vi "Test-Control-Panel.vi"() -> ()   [LabVIEW 2021]
uses:
  Global-Var-Simulator.vi
  Global-Var-OperService.vi
  Global-Var-ControlPanel.vi
panel:
  out "is_simulator_on":bool
  in  "all_alarm_delete_btn":bool
  in  "start_sim":bool
  in  "stop_sim":bool
  in  "shiner_level_ind_L":dbl
  in  "soap_level_ind_L":dbl
  in  "water_level_ind_L":dbl
  in  "download_values_button":bool
  in  "send_values_btn":bool
  in  "process_stop_btn":bool
  in  "fill_shiner_tank_btn":bool
  in  "fill_soap_tank_btn":bool
  in  "fill_water_tank_btn":bool
  out "low_shiner_level_alarm_ind":bool
  out "low_soap_level_alarm_ind":bool
  out "low_water_level_alarm_ind":bool
  out "broken_nozzle_stance_1_alarm_ind":bool
  out "high_temp_tank_1_alarm_ind":bool
  out "high_press_tank_1_alarm_ind":bool
  out "pump_clogged_alarm_ind":bool
  in  "broken_nozzle_stance_1_alarm_btn":bool
  in  "high_temperature_tank_1_alarm_btn":bool
  in  "high_pressure_tank_1_alarm_btn":bool
  in  "pump_clogged_alarm_btn":bool
  out "shiner_tank_L":dbl(slide) scale=0.0..500.0
  out "soap_tank_L":dbl(slide) scale=0.0..500.0
  out "water_tank_L":dbl(slide) scale=0.0..500.0
  # "ON/OFF"
  # "Tank control section"
  # "Alarms control\nand indication"
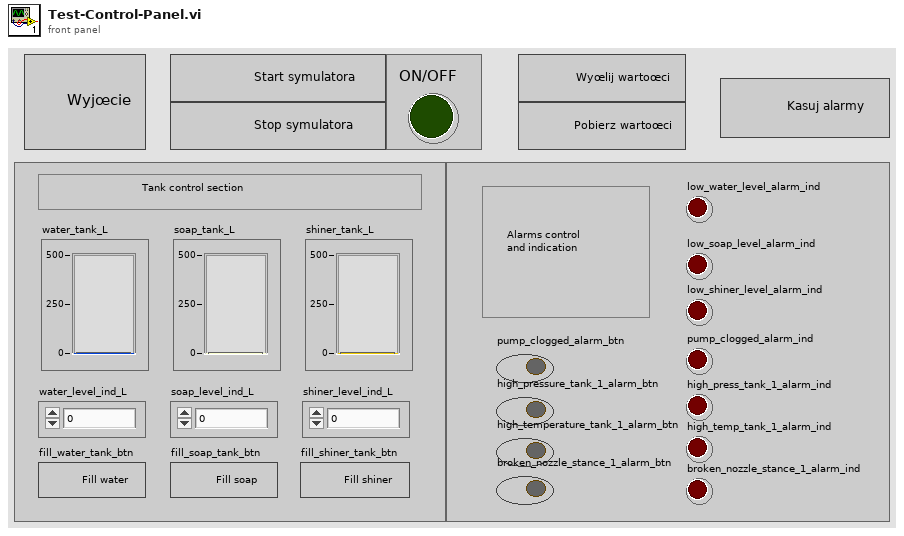
[diagram p1: front panel]
types:
  T1 = enum32{"Invalid", "Standard", "Closed", "Hidden", "Minimized", "Maximized"}
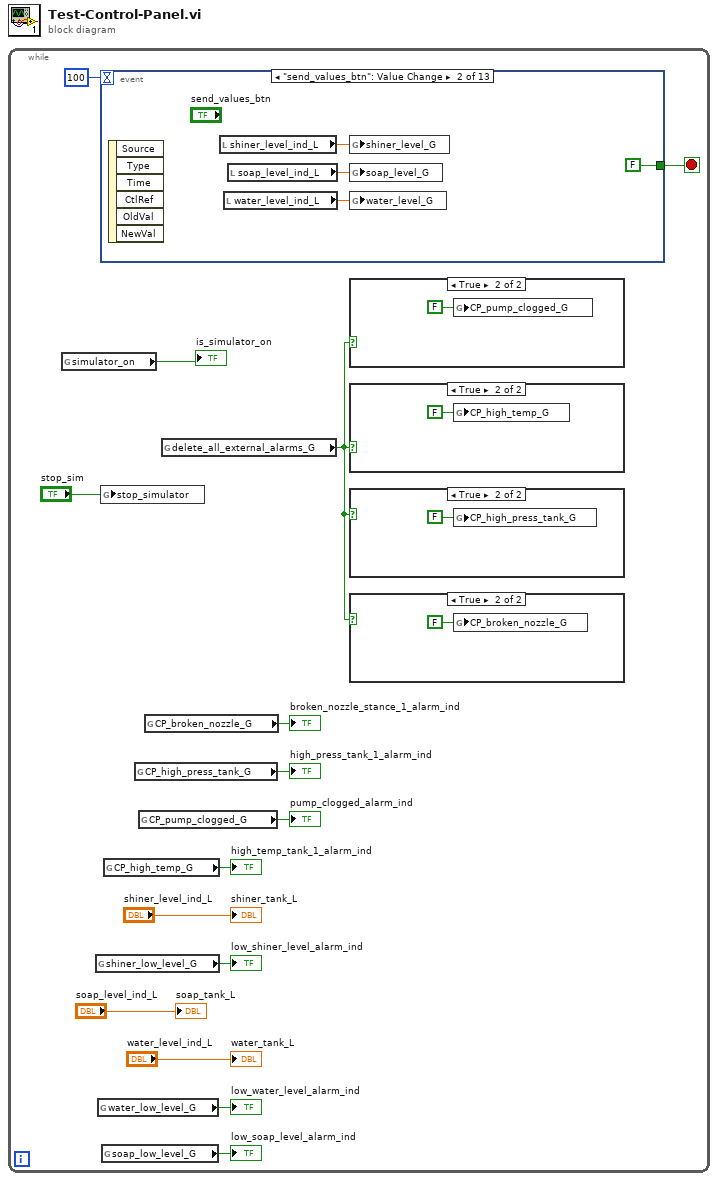
[diagram p0: block diagram]
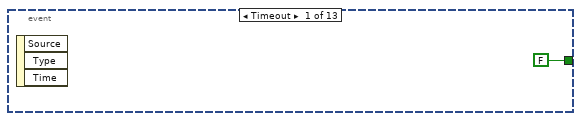
[diagram p6: hidden frame]
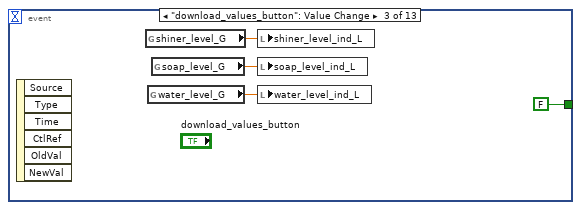
[diagram p7: hidden frame]
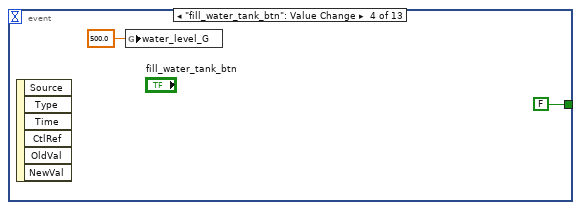
[diagram p8: hidden frame]
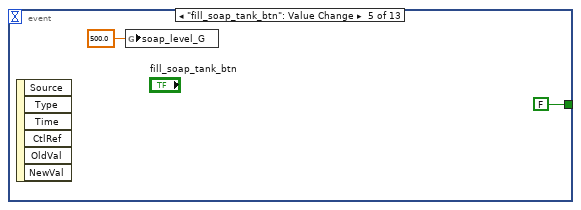
[diagram p9: hidden frame]
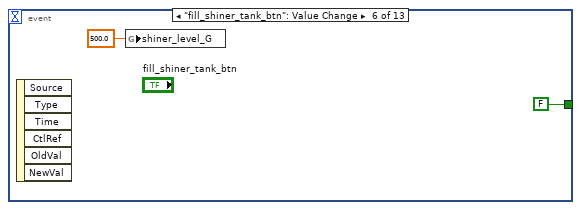
[diagram p10: hidden frame]
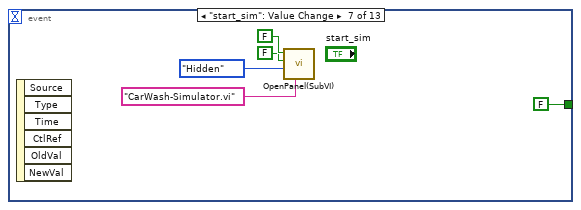
[diagram p11: hidden frame]
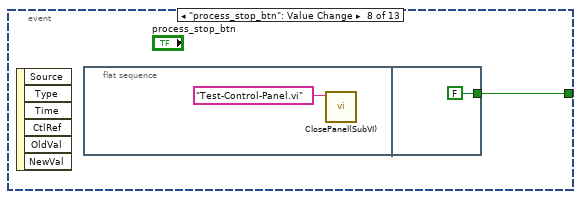
[diagram p12: hidden frame]
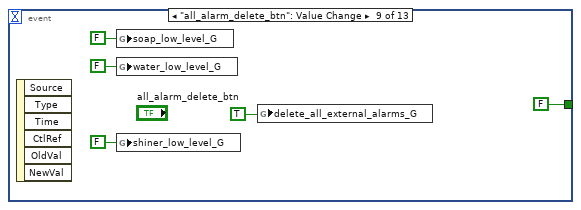
[diagram p13: hidden frame]
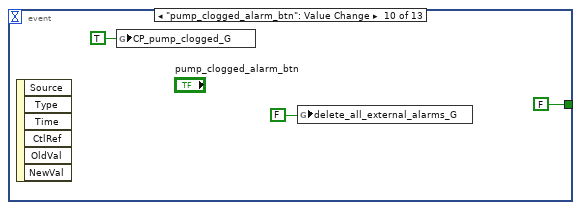
[diagram p14: hidden frame]
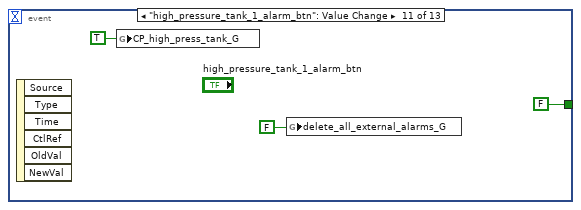
[diagram p15: hidden frame]
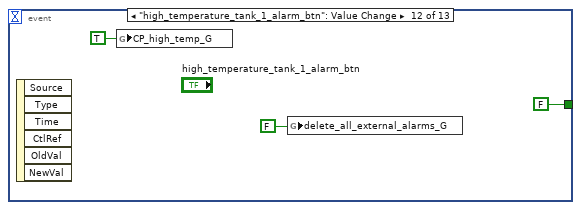
[diagram p16: hidden frame]
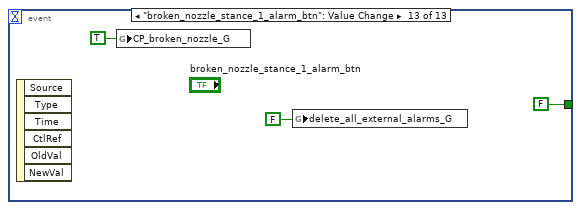
[diagram p17: hidden frame]
diagram:
  n1 = while {
    stop <- w10 stop-if-true
    n2 = global read "Global-Var-Simulator.vi" "simulator_on"() -> (→"is_simulator_on":bool)
    n3 = global read "Global-Var-Simulator.vi" "shiner_low_level_G"() -> (→"low_shiner_level_alarm_ind":bool)
    n4 = global read "Global-Var-Simulator.vi" "water_low_level_G"() -> (→"low_water_level_alarm_ind":bool)
    n5 = event shown="[1] \"send_values_btn\": Value Change" {
      selector: _ -> [_ _ _ _ _ _ _ _ _ _ _ _ _]
      dyn-events: _ -> [_ _ _ _ _ _ _ _ _ _ _ _ _]
      timeout: 100 -> [_ _ _ _ _ _ _ _ _ _ _ _ _]
      tunnel: [FALSE FALSE FALSE FALSE FALSE FALSE FALSE w40 FALSE FALSE FALSE FALSE FALSE] -> w10
      event Timeout {
        n6 = event-data() -> ()  [unwired: 1 in, 3 out]
      }
      event "send_values_btn": Value Change {
        n7 = event-data() -> ()  [unwired: 1 in, 6 out]
        n8 = local read "shiner_level_ind_L"() -> (w22:dbl)
        n9 = local read "water_level_ind_L"() -> (w24:dbl)
        n10 = local read "soap_level_ind_L"() -> (w23:dbl)
        n11 = global write "Global-Var-Simulator.vi" "shiner_level_G"(w22) -> ()
        n12 = global write "Global-Var-Simulator.vi" "soap_level_G"(w23) -> ()
        n13 = global write "Global-Var-Simulator.vi" "water_level_G"(w24) -> ()
      }
      event "download_values_button": Value Change {
        n14 = event-data() -> ()  [unwired: 1 in, 6 out]
        n15 = global read "Global-Var-Simulator.vi" "shiner_level_G"() -> (w28:dbl)
        n16 = global read "Global-Var-Simulator.vi" "water_level_G"() -> (w26:dbl)
        n17 = global read "Global-Var-Simulator.vi" "soap_level_G"() -> (w27:dbl)
        n18 = local write "shiner_level_ind_L"(w28) -> ()
        n19 = local write "soap_level_ind_L"(w27) -> ()
        n20 = local write "water_level_ind_L"(w26) -> ()
      }
      event "fill_water_tank_btn": Value Change {
        n21 = event-data() -> ()  [unwired: 1 in, 6 out]
        n22 = global write "Global-Var-Simulator.vi" "water_level_G"(500.0 ("water_level_G")) -> ()
      }
      event "fill_soap_tank_btn": Value Change {
        n23 = event-data() -> ()  [unwired: 1 in, 6 out]
        n24 = global write "Global-Var-Simulator.vi" "soap_level_G"(500.0 ("soap_level_G")) -> ()
      }
      event "fill_shiner_tank_btn": Value Change {
        n25 = event-data() -> ()  [unwired: 1 in, 6 out]
        n26 = global write "Global-Var-Simulator.vi" "shiner_level_G"(500.0 ("shiner_level_G")) -> ()
      }
      event "start_sim": Value Change {
        n27 = event-data() -> ()  [unwired: 1 in, 6 out]
        n28 = call "OpenPanel(SubVI).vi"("String"="CarWash-Simulator.vi", "State"=T1."Hidden", "Wait Until Done"=FALSE, "Auto Dispose Reference"=FALSE) -> ()  [unwired: 8 in]
      }
      event "process_stop_btn": Value Change {
        n29 = event-data() -> ()  [unwired: 1 in, 6 out]
        n30 = flat-sequence {
          tunnel: [FALSE] -> w40
          frame #0 {
            n31 = call "ClosePanel(SubVI).vi"("String"="Test-Control-Panel.vi") -> ()  [unwired: 11 in]
          }
          frame #1 {
          }
        }
      }
      event "all_alarm_delete_btn": Value Change {
        n32 = event-data() -> ()  [unwired: 1 in, 6 out]
        n33 = global write "Global-Var-Simulator.vi" "soap_low_level_G"(FALSE ("soap_low_level_G")) -> ()
        n34 = global write "Global-Var-Simulator.vi" "water_low_level_G"(FALSE ("water_low_level_G")) -> ()
        n35 = global write "Global-Var-Simulator.vi" "shiner_low_level_G"(FALSE ("shiner_low_level_G")) -> ()
        n36 = global write "Global-Var-OperService.vi" "delete_all_external_alarms_G"(TRUE ("delete_all_external_alarms_G")) -> ()
      }
      event "pump_clogged_alarm_btn": Value Change {
        n37 = event-data() -> ()  [unwired: 1 in, 6 out]
        n38 = global write "Global-Var-ControlPanel.vi" "CP_pump_clogged_G"(TRUE ("CP_pump_clogged_G")) -> ()
        n39 = global write "Global-Var-OperService.vi" "delete_all_external_alarms_G"(FALSE ("delete_all_external_alarms_G")) -> ()
      }
      event "high_pressure_tank_1_alarm_btn": Value Change {
        n40 = event-data() -> ()  [unwired: 1 in, 6 out]
        n41 = global write "Global-Var-ControlPanel.vi" "CP_high_press_tank_G"(TRUE ("CP_high_temp_G")) -> ()
        n42 = global write "Global-Var-OperService.vi" "delete_all_external_alarms_G"(FALSE ("delete_all_external_alarms_G")) -> ()
      }
      event "high_temperature_tank_1_alarm_btn": Value Change {
        n43 = event-data() -> ()  [unwired: 1 in, 6 out]
        n44 = global write "Global-Var-ControlPanel.vi" "CP_high_temp_G"(TRUE ("CP_high_temp_G")) -> ()
        n45 = global write "Global-Var-OperService.vi" "delete_all_external_alarms_G"(FALSE ("delete_all_external_alarms_G")) -> ()
      }
      event "broken_nozzle_stance_1_alarm_btn": Value Change {
        n46 = event-data() -> ()  [unwired: 1 in, 6 out]
        n47 = global write "Global-Var-ControlPanel.vi" "CP_broken_nozzle_G"(TRUE ("CP_broken_nozzle_G")) -> ()
        n48 = global write "Global-Var-OperService.vi" "delete_all_external_alarms_G"(FALSE ("delete_all_external_alarms_G")) -> ()
      }
    }
    n49 = global write "Global-Var-Simulator.vi" "stop_simulator"("stop_sim") -> ()
    n50 = global read "Global-Var-Simulator.vi" "soap_low_level_G"() -> (→"low_soap_level_alarm_ind":bool)
    n51 = global read "Global-Var-ControlPanel.vi" "CP_high_temp_G"() -> (→"high_temp_tank_1_alarm_ind":bool)
    n52 = global read "Global-Var-ControlPanel.vi" "CP_high_press_tank_G"() -> (→"high_press_tank_1_alarm_ind":bool)
    n53 = global read "Global-Var-ControlPanel.vi" "CP_pump_clogged_G"() -> (→"pump_clogged_alarm_ind":bool)
    n54 = global read "Global-Var-ControlPanel.vi" "CP_broken_nozzle_G"() -> (→"broken_nozzle_stance_1_alarm_ind":bool)
    n55 = global read "Global-Var-OperService.vi" "delete_all_external_alarms_G"() -> (w6:bool)
    n56 = case shown="True" w6 {
      frame False {
      }
      frame True {
        n57 = global write "Global-Var-ControlPanel.vi" "CP_pump_clogged_G"(FALSE ("pump_clogged_alarm_btn")) -> ()
      }
    }
    n58 = case shown="True" w6 {
      frame False {
      }
      frame True {
        n59 = global write "Global-Var-ControlPanel.vi" "CP_high_temp_G"(FALSE ("pump_clogged_alarm_btn")) -> ()
      }
    }
    n60 = case shown="True" w6 {
      frame False {
      }
      frame True {
        n61 = global write "Global-Var-ControlPanel.vi" "CP_high_press_tank_G"(FALSE ("pump_clogged_alarm_btn")) -> ()
      }
    }
    n62 = case shown="True" w6 {
      frame False {
      }
      frame True {
        n63 = global write "Global-Var-ControlPanel.vi" "CP_broken_nozzle_G"(FALSE ("pump_clogged_alarm_btn")) -> ()
      }
    }
    "water_tank_L" <- "water_level_ind_L"
    "soap_tank_L" <- "soap_level_ind_L"
    "shiner_tank_L" <- "shiner_level_ind_L"
  }
